vi "FRCts20_Backend_Comment_GET_reform.vi"(7 "Note":T1, 8 "error in (no error)":errorcluster, 11 "recordset data":variant[][](array[variant])) -> (0 "error out":errorcluster, 3 "data string":string)   [LabVIEW 2013, in "FRCts20_Backend_Engine.lvlib"]
doc: "Reforms and returns a specific comment's information"
uses:
  FRCts20_Backend_Engine.lvlib
  FRCts20_Backend_API/FRCts20_Backend_API_Note.ctl
  FRCts20_Backend_DBCluster_Comment_GET.ctl
  <vilib>/addons/database/_DB Variant To Data/Database Variant To Data.xnode
  FRCts20_Backend_API/FRCts20_Backend_API.lvlib
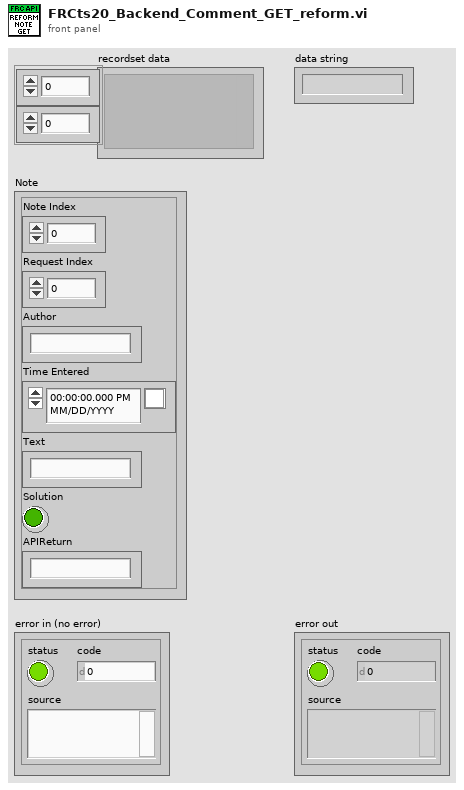
[diagram p1: front panel]
types:
  T1 = typedef "FRCts20_Backend_API.lvlib/FRCts20_Backend_API_Note.ctl" = cluster{"Note Index":u32, "Request Index":u32, "Author":string, "Time Entered":timestamp, "Text":string, "Solution":bool, "APIReturn":string}
  T2 = typedef "FRCts20_Backend_Engine.lvlib/FRCts20_Backend_DBCluster_Comment_GET.ctl" = cluster{"Text":string, "Time Entered":timestamp, "Author":string, "Solution":u16, "ReqNumber":u32}
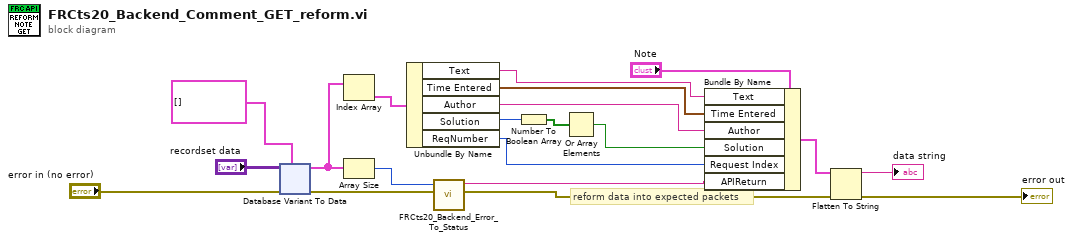
[diagram p0: block diagram]
diagram:
  # "reform data into expected packets"
  n1 = xnode "Database Variant To Data"("database variant"="recordset data", "error in (no error)"="error in (no error)", "type"=T2[] []) -> ("data"=w11:T2[], "error out"=w10:errorcluster)
  n2 = Index Array(array=w11) -> (element=w12:T2)  [unwired: 1 in]
  n3 = Array Size(array=w11) -> (size(s)=w16:i32)
  n4 = Unbundle By Name(w12) -> ("Text"=w13:string, "Time Entered"=w14:timestamp, "Author"=w15:string, "Solution"=w2:u16, "ReqNumber"=w4:u32)
  n5 = call "FRCts20_Backend_Error_To_Status.vi"("error in (no error)"=w10, "rows affected"=w16) -> ("error out"=w17:errorcluster, "String"=w5:string)  [unwired: 8 in]
  n6 = Number To Boolean Array(number=w2) -> (Boolean array=w3:bool[])
  n7 = Or Array Elements(Boolean array=w3) -> (logical OR=w1:bool)
  n8 = Bundle By Name(cluster="Note", "Text"=w13, "Time Entered"=w14, "Author"=w15, "Solution"=w1, "Request Index"=w4, "APIReturn"=w5) -> (w7:T1)
  n9 = Flatten To String(anything=w7, error in (no error)=w17) -> (data string=→"data string":string, error out=→"error out":errorcluster)  [unwired: 2 in, 1 out]
